vi "ShowAfterBuriedPicture.vi"(6 "RedChannel":u8[](array[numeric]), 7 "bottom":i16, 9 "GreenChannel":u8[](array[numeric]), 10 "right":i16, 11 "BlueChannel":u8[](array[numeric])) -> (3 "new picture":picture, 4 "AfterRecombinedData":u8[](array[numeric]))   [LabVIEW 2016]
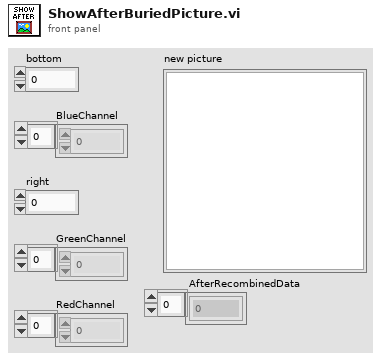
[diagram p1: front panel]
types:
  T1 = typedef "imagedata.ctl" = cluster{"image type":i32, "image depth":i32, "image":u8[], "mask":u8[], "colors":u32[], "Rectangle":cluster{"left":i16, "top":i16, "right":i16, "bottom":i16}}
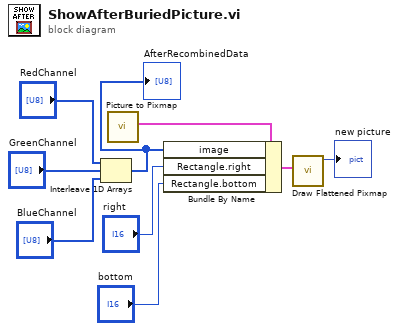
[diagram p0: block diagram]
diagram:
  n1 = Interleave 1D Arrays("RedChannel", "GreenChannel", "BlueChannel") -> (w1:u8[])
  "AfterRecombinedData" <- w1
  n2 = call <vilib>:"Picture to Pixmap.vi"() -> ("image data"=w7:T1)  [unwired: 10 in, 1 out]
  n3 = Bundle By Name(cluster=w7, "image"=w1, "Rectangle.right"="right", "Rectangle.bottom"="bottom") -> (w8:T1)
  n4 = call <vilib>:"Draw Flattened Pixmap.vi"("image data"=w8) -> ("new picture"=→"new picture":picture)  [unwired: 8 in]
